vi "ProcessPOXData.vi"(7 "Application Data":T1, 8 "error in (no error)":errorcluster, 9 "POX Data":string, 11 "Acq Thread Data in":T2) -> (0 "error out":errorcluster)   [LabVIEW 2019]
uses:
  Typedefs/Acquisition Thread/#cluster_AcqThreadData.ctl
  <vilib>/MagicBox/Device/Arduino/Arduino.lvclass
  <vilib>/MagicBox/Peripherals/POX/POX.lvclass
  Typedefs/Acquisition Thread/#enum_AcqThreadState.ctl
  Typedefs/#cluster_GUIRefs.ctl
  Typedefs/#cluster_ApplicationData.ctl
  Typedefs/Acquisition Thread/#cluster_AcqQueueData.ctl
  Typedefs/Acquisition Thread/#enum_AcquisitionTask.ctl
  Typedefs/Saving Thread/#cluster_SavingQueueData.ctl
  Typedefs/Saving Thread/#enum_SavingTask.ctl
  Typedefs/Saving Thread/#cluster_SaveData.ctl
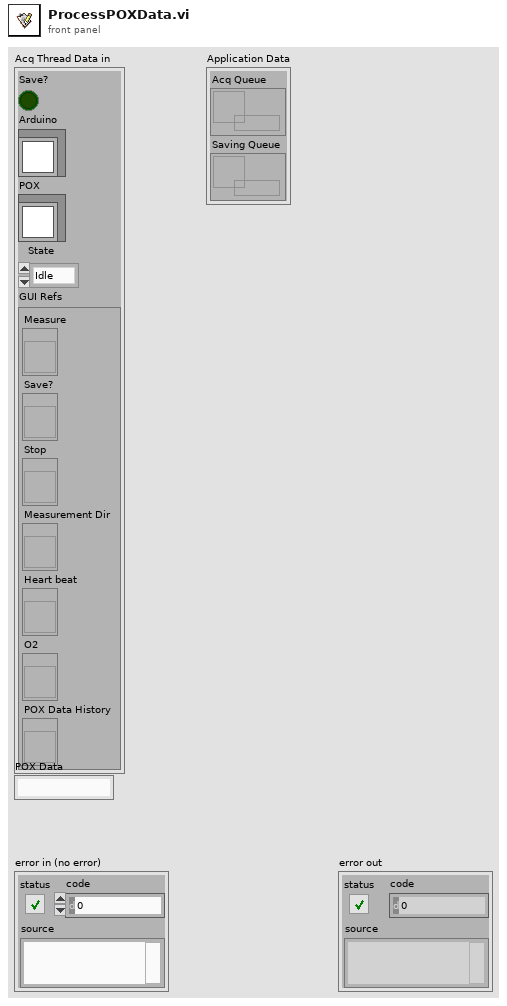
[diagram p1: front panel]
types:
  T1 = typedef "#cluster_ApplicationData.ctl" = cluster{"Acq Queue":refnum<queue>, "Saving Queue":refnum<queue>}
  T2 = typedef "#cluster_AcqThreadData.ctl" = cluster{"Save?":bool, "Arduino":refnum<class "Arduino.lvclass">, "POX":refnum<class "POX.lvclass">, "State":T3, "GUI Refs":T4}
  T3 = typedef "#enum_AcqThreadState.ctl" = enum16{"Idle", "Operate", "Error"}
  T4 = typedef "#cluster_GUIRefs.ctl" = cluster{"Measure":refnum<vi>, "Save?":refnum<vi>, "Stop":refnum<vi>, "Measurement Dir":refnum<vi>, "Heart beat":refnum<vi>, "O2":refnum<vi>, "POX Data History":refnum<vi>}
  T5 = typedef "#cluster_SaveData.ctl" = cluster{"Heart Beat":dbl, "O2":dbl}
  T6 = typedef "#cluster_SavingQueueData.ctl" = cluster{"Task":T7, "Data":variant}
  T7 = typedef "#enum_SavingTask.ctl" = enum16{"Set directory", "Save", "Stop", "Close"}
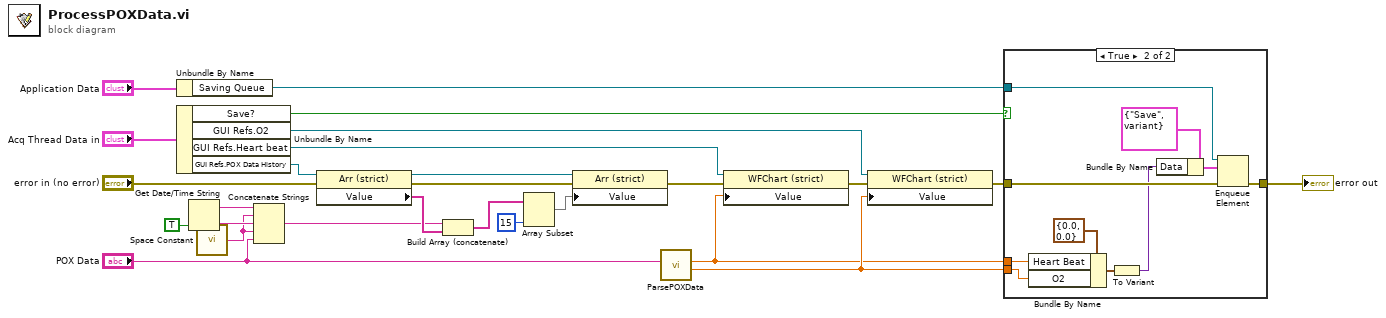
[diagram p0: block diagram]
diagram:
  n1 = Unbundle By Name("Application Data") -> ("Saving Queue"=w18:refnum<queue>)
  n2 = Unbundle By Name("Acq Thread Data in") -> ("Save?"=w16:bool, "GUI Refs.O2"=w20:refnum<vi>, "GUI Refs.Heart beat"=w21:refnum<vi>, "GUI Refs.POX Data History"=w14:refnum<vi>)
  n3 = Get Date/Time String(want seconds? (F)=TRUE) -> (date string=w9:string, time string=w8:string)  [unwired: 2 in]
  n4 = call <vilib>:"Space Constant.vi"() -> ("String"=w7:string)
  n5 = Concatenate Strings(w9, w7, w8, w7, "POX Data") -> (w5:string)
  n6 = property class="Arr (strict)"(reference=w14, error in="error in (no error)") -> (reference out=w13:refnum<vi>, error out=w12:errorcluster, "Value"=w10:string[])
  n7 = Build Array (concatenate)(w5, w10) -> (w4:string[])
  n8 = Array Subset(array=w4, length=15) -> (w3:string[])  [unwired: 1 in]
  n9 = property class="Arr (strict)"(reference=w13, error in=w12, "Value"=w3) -> (error out=w11:errorcluster)  [unwired: 1 out]
  n10 = call "ParsePOXData.vi"("POX Data in"="POX Data") -> ("O2"=w23:dbl, "Hear Beat"=w22:dbl)  [unwired: 8 in, 1 out]
  n11 = property class="WFChart (strict)"(reference=w21, error in=w11, "Value"=w22) -> (error out=w19:errorcluster)  [unwired: 1 out]
  n12 = property class="WFChart (strict)"(reference=w20, error in=w19, "Value"=w23) -> (error out=w17:errorcluster)  [unwired: 1 out]
  n13 = case shown="True" w16 {
    tunnel: w22 -> [_ w34]
    tunnel: w23 -> [_ w33]
    tunnel: w18 -> [_ w36]
    tunnel: w17 -> [w27 w37]
    tunnel: [w27 w28] -> w25
    frame False {
    }
    frame True {
      n14 = Bundle By Name(cluster=T5 {"Heart Beat"=0.0, "O2"=0.0} ("Save Data"), "Heart Beat"=w34, "O2"=w33) -> (w30:T5)
      n15 = To Variant(anything=w30) -> (Variant=w29:variant)
      n16 = Bundle By Name(cluster=T6 {"Task"=enum."Save", "Data"=variant} ("element"), "Data"=w29) -> (w31:T6)
      n17 = Enqueue Element(queue=w36, element=w31, error in (no error)=w37) -> (error out=w28:errorcluster)  [unwired: 1 in, 2 out]
    }
  }
  "error out" <- w25
